vi "Set Sender.vi"(10 "Sender":refnum<class "Sender.lvclass">, 11 "Override Error Msg Strategy in":refnum<class "Override Error Msg Strategy.lvclass">) -> (3 "Override Error Msg Strategy out":refnum<class "Override Error Msg Strategy.lvclass">)   [LabVIEW 2021, in "Override Error Msg Strategy.lvlib" / "Override Error Msg Strategy.lvclass"]
uses:
  Override Error Msg Strategy.lvclass
  Override Error Msg Strategy.lvclass/Override Error Msg Strategy.ctl
  jettl/Sender/Sender/Sender.lvclass
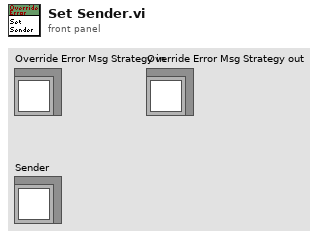
[diagram p1: front panel]
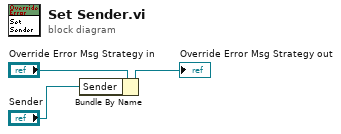
[diagram p0: block diagram]
diagram:
  n1 = Bundle By Name(cluster="Override Error Msg Strategy in", "Sender"="Sender") -> (→"Override Error Msg Strategy out":refnum<class "Override Error Msg Strategy.lvclass">)
